vi "WaveGenerator.vi"(0 "Data array":dbl[][](array[numeric]), 1 "dt":dbl, 3 "TestLoops":i32, 5 "VMIC command":dbl[](array[numeric]), 9 "WaveDefineArray":T1[](array[typedef]) {"Enable" items=["不使能", "使能"]; "Wave" items=["0指令", "正弦波", "方波", "三角波", "常值", "波形数据", "白噪声", "正弦扫频", "梯度加载", "VMIC"]; "ChannelType" items=["标准波形跟踪"=1, "扫频测试"=2, "消除多余力"=3, "梯度加载"=4, "载荷谱跟踪"=5, "模拟输入跟踪"=9]; "ChannelStatus" items=["通道关", "位置通道", "加载通道"]}, 11 "Angle":dbl[](array[numeric]), 12 "AxisForce":dbl[](array[numeric]), 14 "LastVMICcommand":dbl[](array[numeric])) -> (4 "wave out 2":dbl[](array[numeric]), 6 "Command":dbl[](array[numeric]), 10 "Boolean":bool, 13 "VMICafterFilter":dbl[](array[numeric]), 15 "type out":dbl[](array[numeric]))   [LabVIEW 2020]
uses:
  ChannelCommand.ctl
  Control 1.ctl
  WaveType.ctl
  MoterEnable.ctl
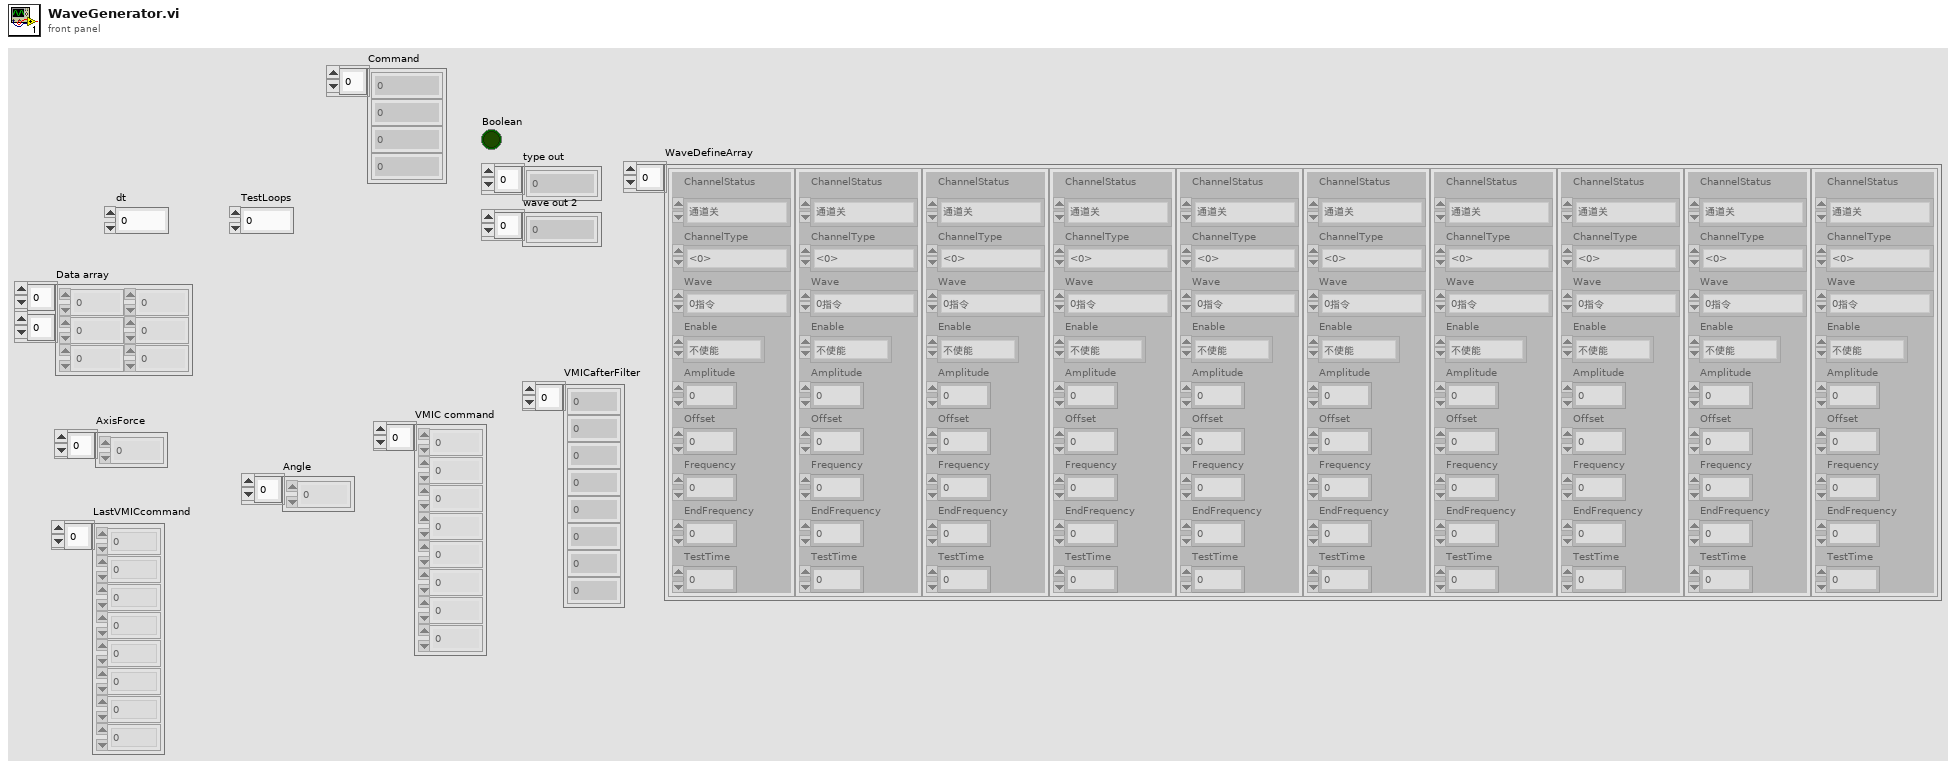
[diagram p1: front panel]
types:
  T1 = typedef "ChannelCommand.ctl" = cluster{"ChannelStatus":T2, "ChannelType":i32, "Wave":T3, "Enable":T4, "Amplitude":dbl, "Offset":dbl, "Frequency":dbl, "EndFrequency":dbl, "TestTime":dbl}
  T2 = typedef "Control 1.ctl" = i32
  T3 = typedef "WaveType.ctl" = i32
  T4 = typedef "MoterEnable.ctl" = u16
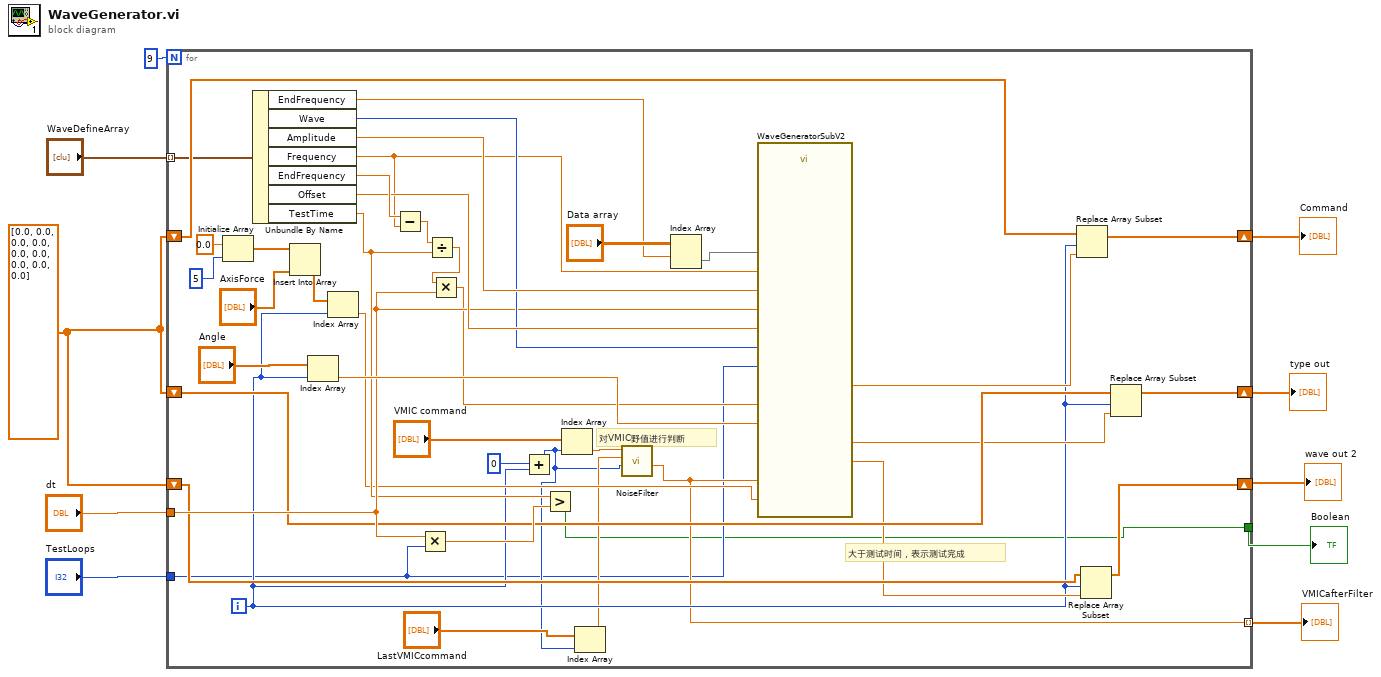
[diagram p0: block diagram]
diagram:
  w4 = dbl[] [0.0, 0.0, 0.0, 0.0, 0.0, 0.0, 0.0, 0.0, 0.0]
  n1 = for {
    N: 9 -> [_]
    tunnel: "dt" -> [w37]
    tunnel: "TestLoops" -> [w12]
    tunnel: "WaveDefineArray" -> [w50] mode=indexing
    shift-right: [w51] -> w7
    shift-left: w4 -> [w52]
    tunnel: [w11] -> w3
    shift-right: [w33] -> w6
    shift-left: w4 -> [w32]
    shift-right: [w30] -> w5
    shift-left: w4 -> [w29]
    tunnel: [w13] -> w1 mode=indexing
    i -> [w19]
    # "对VMIC野值进行判断"
    # "大于测试时间，表示测试完成"
    n2 = Initialize Array(0.0 ("元素"), 5 ("维数大小")) -> (w22:dbl[])
    n3 = Unbundle By Name(w50) -> ("EndFrequency"=w48:dbl, "Wave"=w41:T3, "Amplitude"=w43:dbl, "Frequency"=w35:dbl, "EndFrequency"=w47:dbl, "Offset"=w42:dbl, "TestTime"=w34:dbl)
    n4 = Insert Into Array(array=w22, new element="AxisForce") -> (w21:dbl[])  [unwired: 1 in]
    n5 = Index Array(array="Angle", index=w19) -> (element=w39:dbl)
    n6 = Index Array(array=w21, index=w19) -> (element=w20:dbl)
    n7 = Subtract(x=w47, y=w35) -> (x-y=w46:dbl)
    n8 = Multiply(x=w37, y=w12) -> (x*y=w36:dbl)
    n9 = Divide(x=w46, y=w34) -> (x/y=w45:dbl)
    n10 = Multiply(x=w45, y=w37) -> (x*y=w26:dbl)
    n11 = Add(x=0, y=w19) -> (x+y=w14:i32)
    n12 = Greater?(x=w34, y=w36) -> (0:w11:bool)
    n13 = Index Array(array="VMIC command", index=w14) -> (element=w16:dbl)
    n14 = Index Array(array="LastVMICcommand", index=w14) -> (element=w15:dbl)
    n15 = call "NoiseFilter.vi"("loop"=w14, "lastCom"=w15, "TemCom"=w16) -> ("VmicOut"=w13:dbl)  [unwired: 8 in]
    n16 = Index Array(array="Data array", index (row)=w48) -> (element=w44:dbl[])  [unwired: 1 in]
    n17 = call "WaveGeneratorSubV2.vi"("Amplitude"=w43, "Wave"=w41, "ForceSample"=w20, "Data array"=w44, "Frequent"=w35, "Angle"=w39, "Offset"=w42, "deltaF"=w26, "VMIC"=w13, "dt"=w37, "TestLoops"=w12) -> ("Output"=w38:dbl, "Output 2"=w31:dbl, "waveout 3"=w28:dbl)  [unwired: 2 in]
    n18 = Replace Array Subset "Replace Array Subset"(array=w52, new element=w38, index=w19) -> (w51:dbl[])
    n19 = Replace Array Subset "Replace Array Subset"(array=w29, new element=w28, index=w19) -> (w30:dbl[])
    n20 = Replace Array Subset "Replace Array Subset"(array=w32, new element=w31, index=w19) -> (w33:dbl[])
  }
  "Command" <- w7
  "Boolean" <- w3
  "type out" <- w6
  "wave out 2" <- w5
  "VMICafterFilter" <- w1
